vi "Set Slave Address.vi"(8 "error in":errorcluster, 11 "Red-y Read Write CFG in":refnum<class "Red-y Read Write CFG.lvclass">) -> (0 "error out":errorcluster, 3 "Red-y Read Write CFG out":refnum<class "Red-y Read Write CFG.lvclass">)   [LabVIEW 2023, in "Red-y Read Write CFG.lvclass"]
uses:
  Red-y Read Write CFG.lvclass
  Configuration/Configuration JSON/Configuration JSON Base/CFG JSON.lvclass/CFG JSON.ctl
  Red-y Read Write CFG.lvclass/Red-y Read Write CFG.ctl
  804d9e6d-375f-4434-84c9-52b1ea40b60b.vi
  <vilib>/JDP Science/JSONtext/Find Item.vi
  <vilib>/JDP Science/JSONtext/Next JSON Value.vi
  <vilib>/JDP Science/JSONtext/String Subset.vi
  <vilib>/JDP Science/JSONtext/Parsing/Advance past next JSON Value (inlined COPY).vi
  <vilib>/JDP Science/JSONtext/Parsing/Advance past whitespace.vi
  <vilib>/JDP Science/JSONtext/Parsing/Advance past String.vi
  <vilib>/JDP Science/JSONtext/Parsing/Advance past Number.vi
  <vilib>/JDP Science/JSONtext/Parsing/Advance past Line Ending.vi
  <vilib>/JDP Science/JSONtext/Parsing/Parse Full Path or Item Name.vi
  <vilib>/JDP Science/JSONtext/Parsing/Advance past Array.vi
  <vilib>/JDP Science/JSONtext/Parsing/Advance past Object.vi
  <vilib>/JDP Science/JSONtext/support/Error Cluster From Code.vi
  <vilib>/JDP Science/JSONtext/Offset/Find Item Locations by Path.vi
  <vilib>/JDP Science/JSONtext/JSON text to Variant.vi
  <vilib>/Utility/error.llb/Error Cluster From Error Code.vi
  Voegtlin_NI_SMART_Modbus_Drivers/Low Level Driver/Modbus Write U16.vi
  <vilib>/JDP Science/JSONtext/LVClass Serializer/JSONtext LVClass Serializer.lvclass
  <vilib>/ErrorRing/Error Ring.xnode
  Configuration/Configuration JSON/Configuration JSON Base/CFG JSON.lvclass
  Voegtlin_NI_SMART_Modbus_Drivers/Voegtlin_NI_SMART_Modbus_Drivers.lvlib
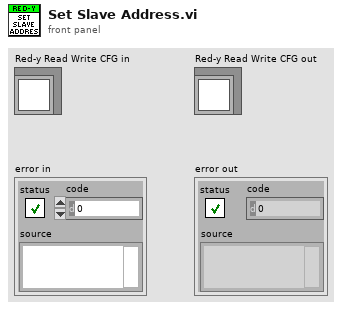
[diagram p1: front panel]
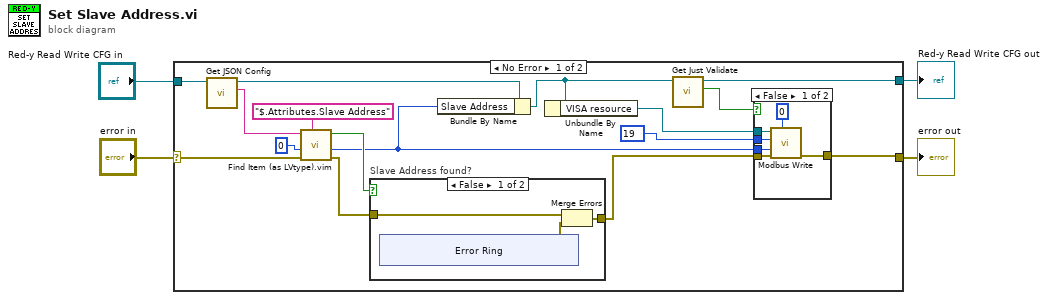
[diagram p0: block diagram]
diagram:
  n1 = case shown="No Error" "error in" {
    selector: "error in" -> [w18 w37]
    tunnel: "Red-y Read Write CFG in" -> [w20 w38]
    tunnel: [w6 w38] -> w3
    tunnel: [w11 w37] -> w2
    frame No Error {
      n2 = call "Get JSON Config.vi"("CFG Base in"=w20) -> ("<JSON>Config>"=w19:string, "CFG Base out"=w10:refnum<class "Red-y Read Write CFG.lvclass">)  [unwired: 9 in]
      n3 = call "Find Item (as LVtype).vim"("$Path or Item Name"="$.Attributes.Slave Address", "error in (no error)"=w18, "Data Type and Default Value"=u16 0, "JSON"=w19) -> ("error out"=w14:errorcluster, "Data"=w9:u16, "Found"=w15:bool)  [unwired: 4 in, 1 out]
      n4 = case "Slave Address found?" shown="False" w15 {
        tunnel: w14 -> [w29 w36]
        tunnel: [w28 w36] -> w13
        frame False {
          n5 = xnode "Error Ring"() -> ("error out"=w30:errorcluster)
          n6 = Merge Errors(w29, w30) -> (w28:errorcluster)
        }
        frame True {
        }
      }
      n7 = Bundle By Name(cluster=w10, "Slave Address"=w9) -> (w8:refnum<class "Red-y Read Write CFG.lvclass">)
      n8 = Unbundle By Name(w8) -> ("VISA resource"=w7:refnum<visa-resource-name>)
      n9 = call "Get Just Validate.vi"("CFG JSON Base in"=w8) -> ("Just Validate"=w5:bool, "CFG JSON Base out"=w6:refnum<class "Red-y Read Write CFG.lvclass">)  [unwired: 9 in]
      n10 = case shown="False" w5 {
        tunnel: w13 -> [w26 w27]
        tunnel: u16 19 -> [w25 _]
        tunnel: [w24 w27] -> w11
        tunnel: w9 -> [w23 _]
        tunnel: w7 -> [w22 _]
        frame False {
          n11 = call-poly "Modbus Write.vi"("Slave Address"=u8 0, "error in (no error)"=w26, "Input data U16"=w23, "Register Start Address"=w25, "VISA resource in"=w22) -> ("error out"=w24:errorcluster)  [unwired: 5 in, 1 out]
        }
        frame True {
        }
      }
    }
    frame Error {
    }
  }
  "error out" <- w2
  "Red-y Read Write CFG out" <- w3
